vi "LogSingleTimeDomain.vi"(5 "TimeDomainVal":dbl[](array[numeric]), 7 "TimeDomainCount":u32[](array[numeric]), 8 "error in":errorcluster, 10 "Cal":T1 {"Downshift_dset" format="%.0x"; "DeltaPhase_dset" format="%.0x"; "Phase_dset" format="%.0x"; "SNR_dset" format="%.0x"; "df_dset" format="%.0x"; "PeakLoc_dset" format="%.0x"; "MaxValue_dset" format="%.0x"; "TImeStamp_dset" format="%.0x"; "TimeString_dset" format="%.0x"}) -> (0 "error out":errorcluster)   [LabVIEW 2018]
uses:
  <vilib>/addons/h5labview2/dataset/H5D.lvlib
  <vilib>/addons/h5labview2/base/H5Equery.vi
  lib_path_mod_20200519.vi
  <vilib>/addons/h5labview2/dataset/H5Dwrite.llb/H5Dwrite.xnode
  <vilib>/addons/h5labview2/space/H5S.lvlib
  HDF5_Tone_refs.ctl
  <vilib>/addons/h5labview2/base/hid_t.ctl
panel:
  out "CountSize":i32
  out "ValSize":i32
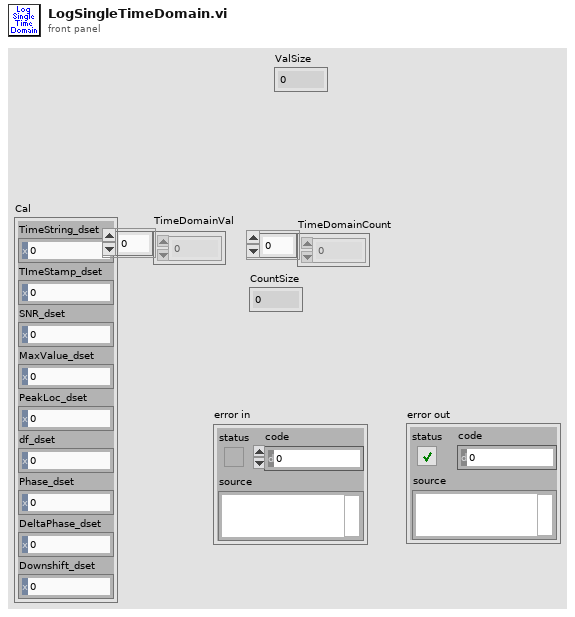
[diagram p1: front panel]
types:
  T1 = typedef "HDF5_Tone_refs.ctl" = cluster{"TimeString_dset":T2, "TImeStamp_dset":T2, "SNR_dset":T2, "MaxValue_dset":T2, "PeakLoc_dset":T2, "df_dset":T2, "Phase_dset":T2, "DeltaPhase_dset":T2, "Downshift_dset":T2}
  T2 = typedef "hid_t.ctl" = i32
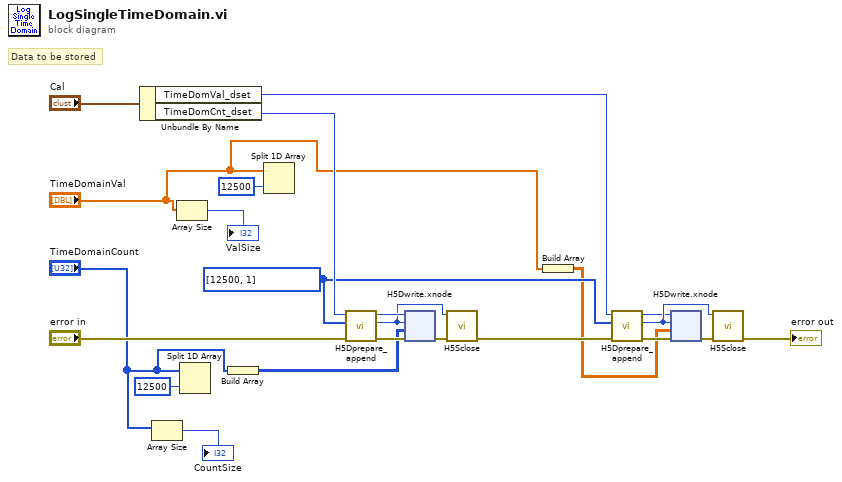
[diagram p0: block diagram]
diagram:
  w9 = u64[] [12500, 1] ("append dims")
  # "Data to be stored"
  n1 = Unbundle By Name("Cal") -> ("TimeDomVal_dset"=w22:T2, "TimeDomCnt_dset"=w23:T2)
  n2 = Array Size(array="TimeDomainCount") -> (size(s)=→"CountSize":i32)
  n3 = Array Size(array="TimeDomainVal") -> (size(s)=→"ValSize":i32)
  n4 = Split 1D Array(array="TimeDomainCount", index=12500) -> ()  [unwired: 2 out]
  n5 = Build Array("TimeDomainCount") -> (w11:u32[][])
  n6 = Split 1D Array(array="TimeDomainVal", index=12500) -> ()  [unwired: 2 out]
  n7 = call <vilib>:"H5Dprepare_append.vi"("error in (no error)"="error in", "append dims"=w9, "dset in"=w23) -> ("error out"=w14:errorcluster, "space out"=w12:T2, "dset out"=w13:T2)  [unwired: 5 in, 1 out]
  n8 = xnode "H5Dwrite.xnode"("error in (no error)"=w14, "data"=w11, "file space"=w12, "ref in"=w13) -> ("error out"=w15:errorcluster)  [unwired: 3 in, 2 out]
  n9 = call <vilib>:"H5Sclose.vi"("error in (no error)"=w15, "space in"=w12) -> ("error out"=w21:errorcluster)  [unwired: 9 in]
  n10 = Build Array("TimeDomainVal") -> (w7:dbl[][])
  n11 = call <vilib>:"H5Dprepare_append.vi"("error in (no error)"=w21, "append dims"=w9, "dset in"=w22) -> ("error out"=w18:errorcluster, "space out"=w20:T2, "dset out"=w19:T2)  [unwired: 5 in, 1 out]
  n12 = xnode "H5Dwrite.xnode"("error in (no error)"=w18, "data"=w7, "file space"=w20, "ref in"=w19) -> ("error out"=w17:errorcluster)  [unwired: 3 in, 2 out]
  n13 = call <vilib>:"H5Sclose.vi"("error in (no error)"=w17, "space in"=w20) -> ("error out"=→"error out":errorcluster)  [unwired: 9 in]
